vi "74HC151.vi"(0 "D 0":bool, 1 "D 1":bool, 2 "D 2":bool, 3 "D 3":bool, 4 "D 4":bool, 5 "D 5":bool, 6 "D 6":bool, 7 "D 7":bool, 8 "A0":bool, 10 "A1":bool, 11 "EN":bool, 12 "A2":bool) -> (23 "布尔":bool)   [LabVIEW 2018]
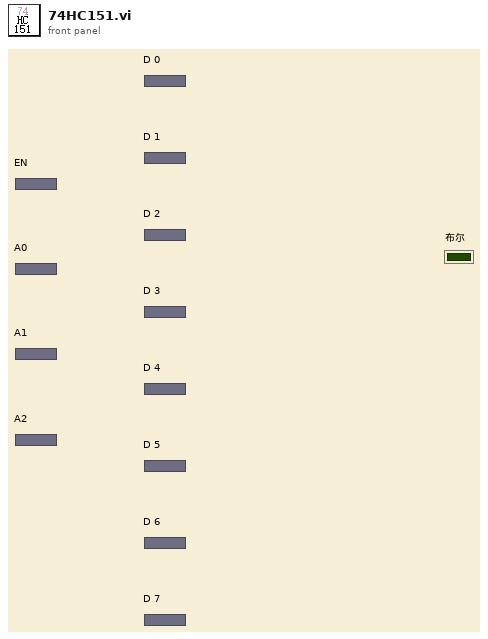
[diagram p1: front panel]
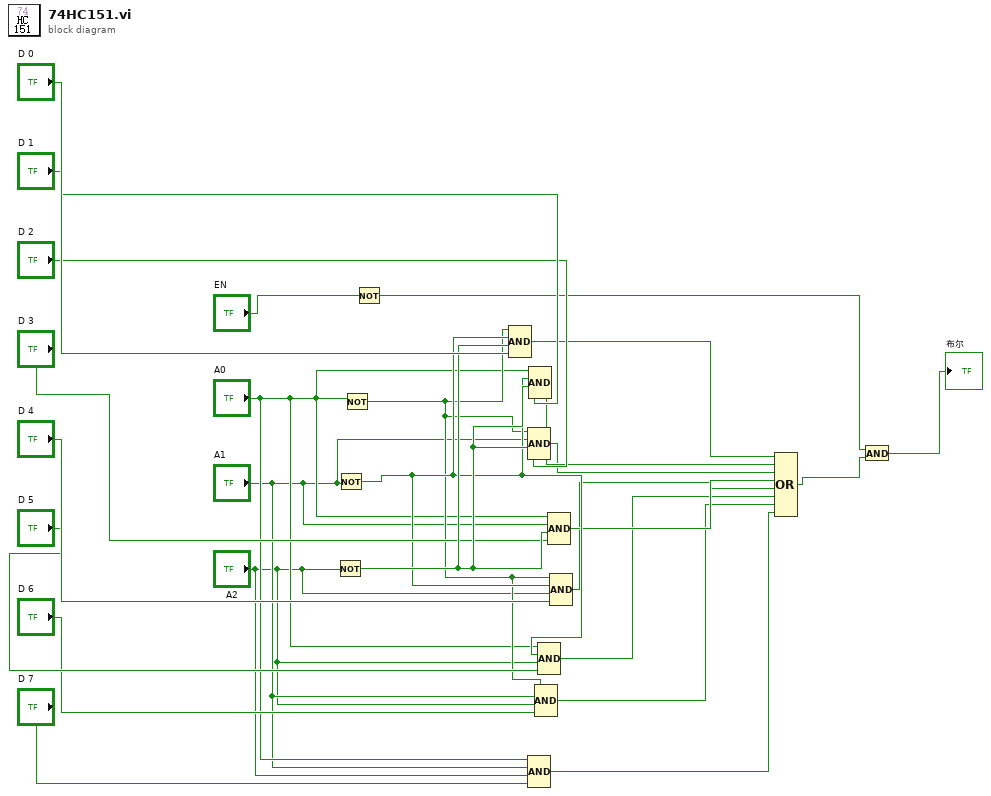
[diagram p0: block diagram]
diagram:
  n1 = Not(x="A2") -> (.not. x?=w23:bool)
  n2 = Not(x="A1") -> (.not. x?=w20:bool)
  n3 = Not(x="A0") -> (.not. x?=w18:bool)
  n4 = Not(x="EN") -> (.not. x?=w1:bool)
  n5 = Compound Arithmetic op=AND ("复合运算")(w18, w20, w23, "D 0") -> (w12:bool)
  n6 = Compound Arithmetic op=AND ("复合运算")(w18, "A1", w23, "D 2") -> (w10:bool)
  n7 = Compound Arithmetic op=AND ("复合运算")("A0", "A1", "A2", "D 7") -> (w5:bool)
  n8 = Compound Arithmetic op=AND ("复合运算")("A0", w20, w23, "D 1") -> (w11:bool)
  n9 = Compound Arithmetic op=AND ("复合运算")(w18, "A1", "A2", "D 6") -> (w6:bool)
  n10 = Compound Arithmetic op=AND ("复合运算")("A0", w20, "A2", "D 5") -> (w7:bool)
  n11 = Compound Arithmetic op=AND ("复合运算")("A0", "A1", w23, "D 3") -> (w9:bool)
  n12 = Compound Arithmetic op=AND ("复合运算")(w18, w20, "A2", "D 4") -> (w8:bool)
  n13 = Compound Arithmetic op=OR ("复合运算")(w12, w11, w10, w9, w8, w7, w6, w5) -> (w4:bool)
  n14 = And(x=w1, y=w4) -> (x .and. y?=→"布尔":bool)
